vi "RTS Get Sorted Filename Index.vi"(6 "Base File Name":string, 8 "Error In":errorcluster, 11 "stripped path":path) -> (0 "Error Out":errorcluster, 1 "Sorted Filename index":i32[](array[numeric]), 3 "filenames":string[](array[string]))   [LabVIEW 2016]
uses:
  <vilib>/Utility/error.llb/whitespace.ctl
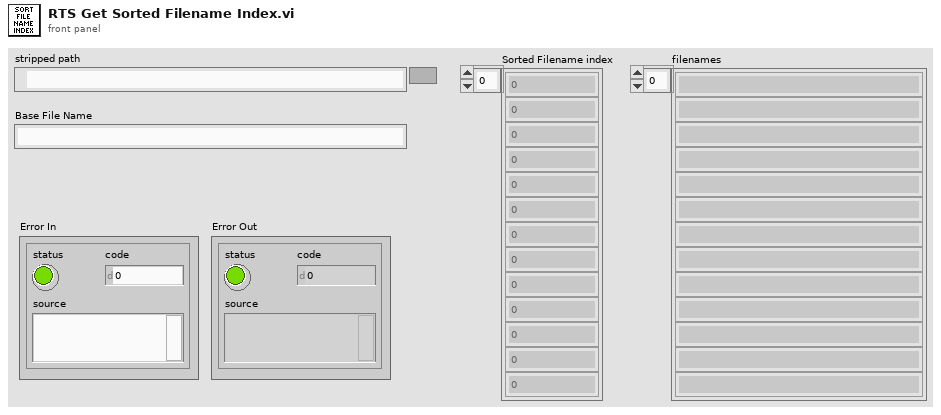
[diagram p1: front panel]
types:
  T1 = typedef "whitespace.ctl" = u16
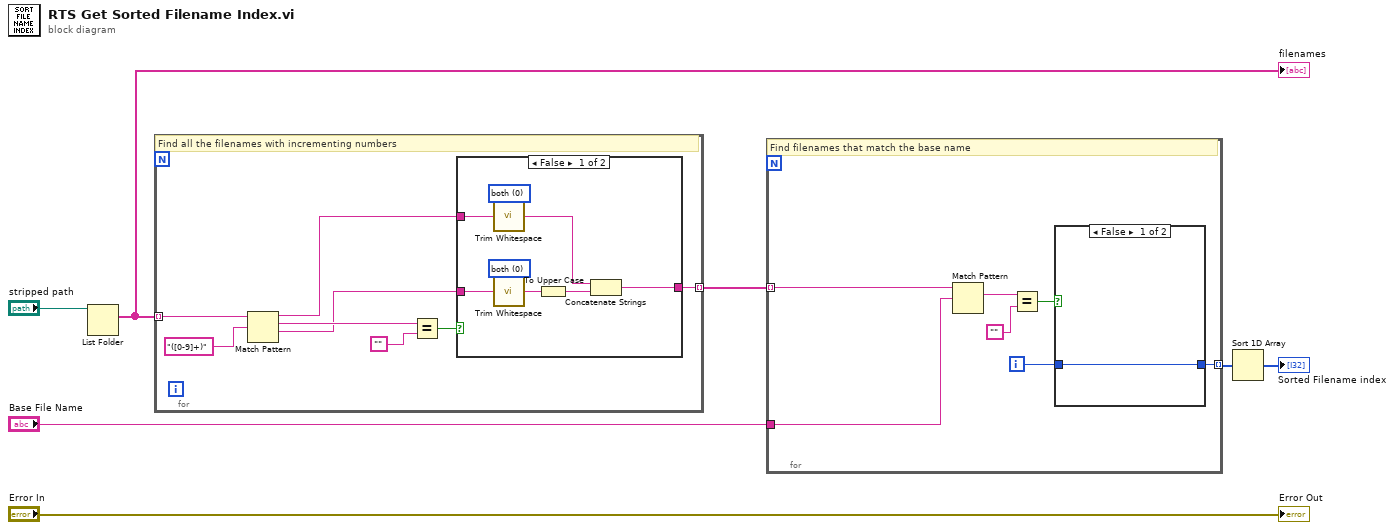
[diagram p0: block diagram]
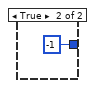
[diagram p2: hidden frame]
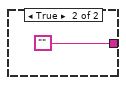
[diagram p3: hidden frame]
diagram:
  n1 = List Folder(path="stripped path") -> (filenames=w4:string[])  [unwired: 3 in, 3 out]
  "filenames" <- w4
  n2 = for {
    tunnel: w4 -> [w14] mode=indexing
    tunnel: [w8] -> w2 mode=indexing
    # "Find all the filenames with incrementing numbers"
    n3 = Match Pattern(string=w14, regular expression="([0-9]+)") -> (before substring=w11:string, match substring=w10:string, after substring=w9:string)  [unwired: 1 in, 1 out]
    n4 = Equal?(x=w10, y="") -> (x = y?=w12:bool)
    n5 = case shown="False" w12 {
      tunnel: w11 -> [w23 _]
      tunnel: w9 -> [w19 _]
      tunnel: [w18 ""] -> w8
      frame False {
        w20 = T1 0 items=["both", "start of string", "end of string"] ("location (both)")
        w21 = T1 0 items=["both", "start of string", "end of string"] ("location (both)")
        n6 = call <vilib>:"Trim Whitespace.vi"("string"=w23, "location (both)"=w21) -> ("trimmed string"=w22:string)
        n7 = call <vilib>:"Trim Whitespace.vi"("string"=w19, "location (both)"=w20) -> ("trimmed string"=w17:string)
        n8 = To Upper Case(1:w17) -> (0:w16:string)
        n9 = Concatenate Strings(w22, w16) -> (w18:string)
      }
      frame True {
      }
    }
  }
  n10 = for {
    tunnel: w2 -> [w31] mode=indexing
    tunnel: "Base File Name" -> [w30]
    tunnel: [w26] -> w3 mode=indexing
    i -> [w27]
    # "Find filenames that match the base name"
    n11 = Match Pattern(string=w31, regular expression=w30) -> (match substring=w25:string)  [unwired: 1 in, 3 out]
    n12 = Equal?(x=w25, y="") -> (x = y?=w28:bool)
    n13 = case shown="False" w28 {
      tunnel: w27 -> [w32 _]
      tunnel: [w32 -1] -> w26
      frame False {
      }
      frame True {
      }
    }
  }
  n14 = Sort 1D Array(array=w3) -> (sorted array=→"Sorted Filename index":i32[])
  "Error Out" <- "Error In"
